vi "Read ChannelOn.vi"(8 "error in (no error)":errorcluster, 11 "T560Output in":refnum<class "T560Output.lvclass">) -> (0 "error out":errorcluster, 2 "ChannelOn":bool, 3 "T560Output out":refnum<class "T560Output.lvclass">)   [LabVIEW 2020, in "T560Output.lvclass"]
uses:
  T560Output.lvclass
  T560Output.lvclass/T560Output.ctl
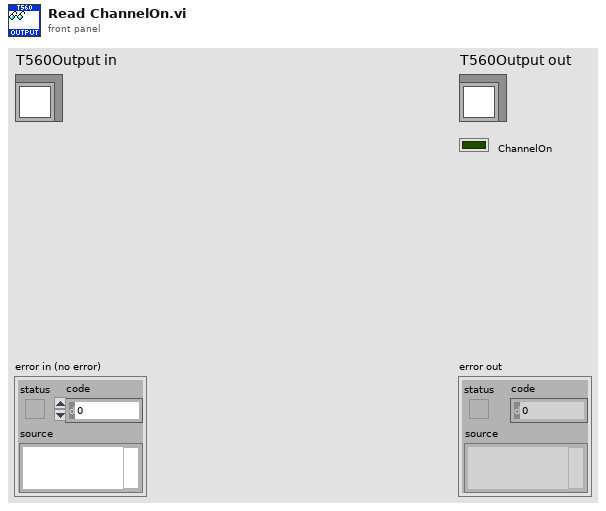
[diagram p1: front panel]
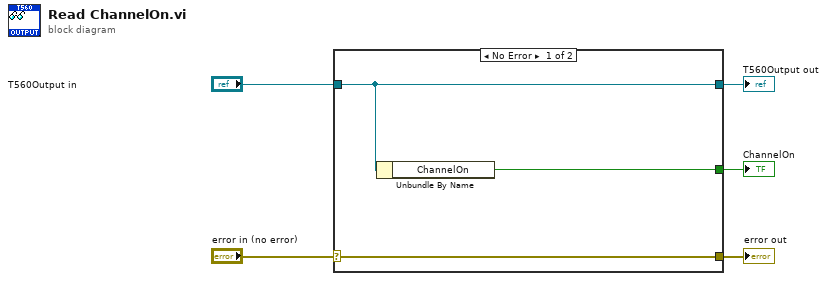
[diagram p0: block diagram]
diagram:
  n1 = case shown="No Error" "error in (no error)" {
    selector: "error in (no error)" -> [w8 w9]
    tunnel: [w8 w9] -> w4
    tunnel: [w7 w10] -> w2
    tunnel: "T560Output in" -> [w7 w10]
    tunnel: [w6 _] -> w1
    frame No Error {
      n2 = Unbundle By Name(w7) -> ("ChannelOn"=w6:bool)
    }
    frame Error {
    }
  }
  "error out" <- w4
  "T560Output out" <- w2
  "ChannelOn" <- w1
